vi "Draw All Joints.vi"(6 "Color":u32(colorbox)=16711680, 7 "Include Inferred Joints?":bool=TRUE, 8 "error in (no error)":errorcluster, 9 "Body Index":i32, 11 "Image":T1) -> (0 "error out":errorcluster, 3 "Image Out":T1)   [LabVIEW 2014, in "LVH-KinectOne.lvlib"]
uses:
  LVH-KinectOne.lvlib
  <vilib>/vision/Image Controls.llb/IMAQ Image.ctl
  Type Defs/JointType.ctl
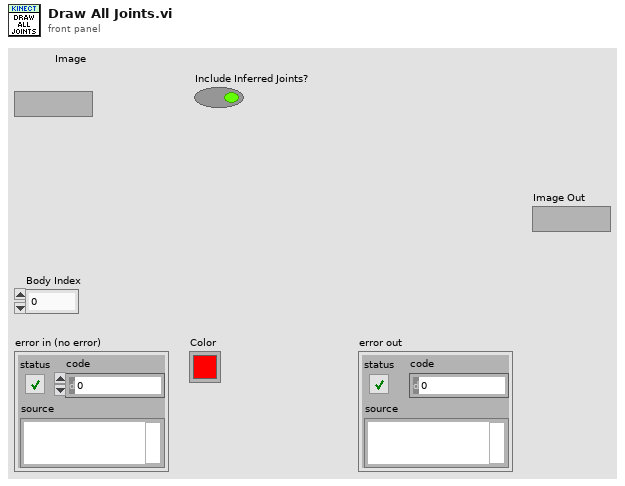
[diagram p1: front panel]
types:
  T1 = typedef "IMAQ Image.ctl" = refnum<image>
  T2 = typedef "LVH-KinectOne.lvlib/JointType.ctl" = i32
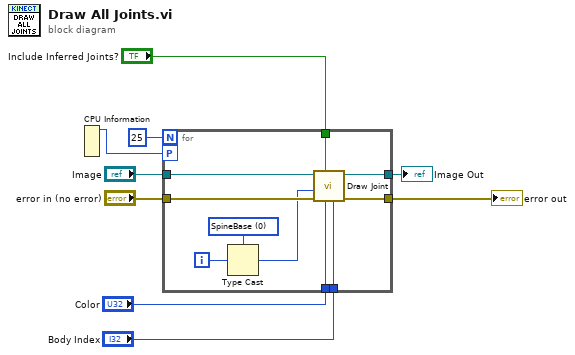
[diagram p0: block diagram]
diagram:
  n1 = CPU Information() -> (4:w3:i32)  [unwired: 3 out]
  n2 = for {
    N: 25 -> [_]
    tunnel: "Image" -> [w15]
    tunnel: [w14] -> w5
    tunnel: "Color" -> [w12]
    workers-P: w3 -> [_]
    tunnel: "Include Inferred Joints?" -> [w11]
    tunnel: "error in (no error)" -> [w16]
    tunnel: [w17] -> w6
    tunnel: "Body Index" -> [w10]
    i -> [w19]
    w18 = T2 0 items=["SpineBase", "SpineMid", "Neck", "Head", "ShoulderLeft", "ElbowLeft", "WristLeft", "HandLeft", "ShoulderRight", "ElbowRight", "WristRight", "HandRight", "HipLeft", "KneeLeft", "AnkleLeft", "FootLeft", "HipRight", "KneeRight", "AnkleRight", "FootRight", "SpineShoulder", "HandTipLeft", "ThumbLeft", "HandTipRight", "ThumbRight"] ("JointType")
    n3 = Type Cast(type=w18, x=w19) -> (*(type *) &x=w13:T2)
    n4 = call "Draw Joint.vi"("Body Index"=w10, "Color"=w12, "Include Inferred Joints?"=w11, "error in"=w16, "JointType"=w13, "Image"=w15) -> ("error out"=w17:errorcluster, "Image Out"=w14:T1)  [unwired: 4 in]
  }
  "error out" <- w6
  "Image Out" <- w5
